vi "AWG Start Pulses.vi"(8 "error in (no error)":errorcluster, 10 "T [s] (1ms)":dbl=0.001, 11 "awg session in":T1) -> (0 "error out":errorcluster, 3 "awg session out":T1)   [LabVIEW 2013, in "AWG.lvlib"]
doc: "AWG wrapper: Starts infinite pulse train with given period."
uses:
  AWG.lvlib
  AWG Session.ctl
  AWG Type.ctl
  Agilent 33XXX Series/Agilent 33XXX Series.lvlib
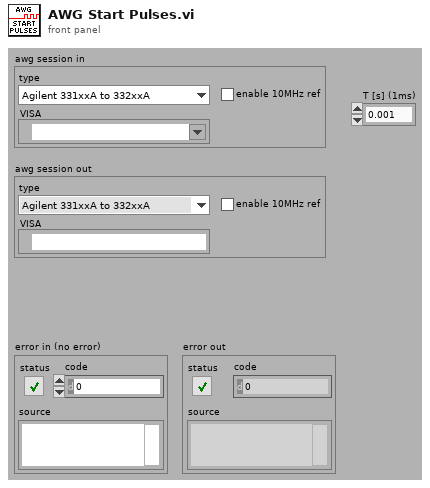
[diagram p1: front panel]
types:
  T1 = typedef "AWG.lvlib/AWG Session.ctl" = cluster{"type":T2, "VISA":refnum<visa-resource-name>, "enable 10MHz ref":bool}
  T2 = typedef "AWG.lvlib/AWG Type.ctl" = enum16{"Agilent 331xxA to 332xxA", "Agilent 335xxA to 336xxA", "dummy"}
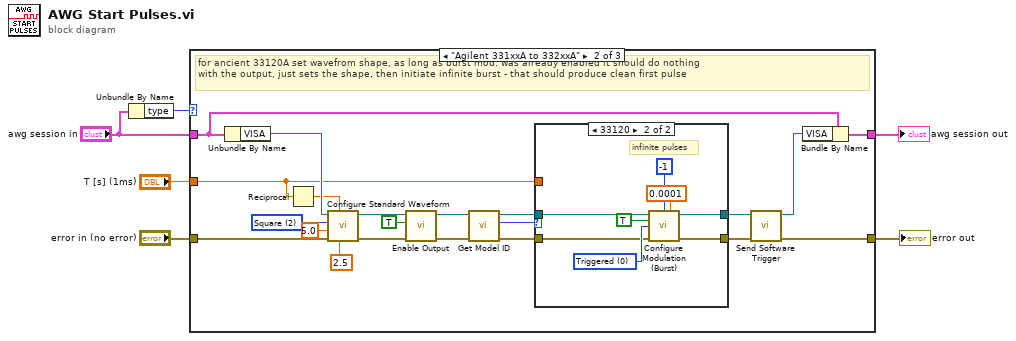
[diagram p0: block diagram]
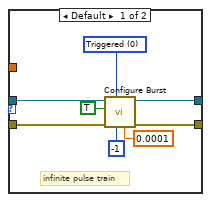
[diagram p3: hidden frame]
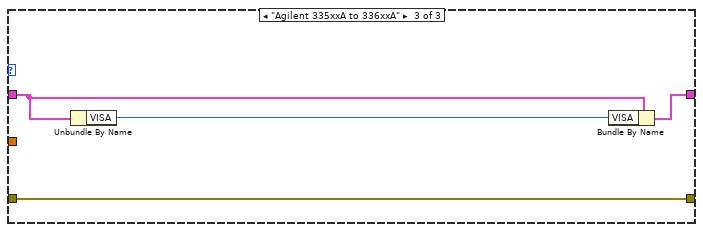
[diagram p4: hidden frame]
diagram:
  n1 = Unbundle By Name("awg session in") -> ("type"=w6:T2)
  n2 = case shown="\"Agilent 331xxA to 332xxA\"" w6 {
    tunnel: "error in (no error)" -> [w8 w20 w46]
    tunnel: [w8 w27 w46] -> w4
    tunnel: "awg session in" -> [w7 w28 w49]
    tunnel: [w7 w29 w48] -> w2
    tunnel: "T [s] (1ms)" -> [_ w9 _]
    frame Default {
    }
    frame "Agilent 331xxA to 332xxA" {
      w23 = u16 2 items=["DC", "Sine", "Square", "Triangle", "Ramp", "Pulse", "Noise", "Sinc", "Negative Ramp", "Exponential Rise", "Exponential Fall", "Cardiac"] ("Waveform Function (1: Sine)")
      # "for ancient 33120A set wavefrom shape, as long as burst mod. was already enabled it should do nothing\nwith the output, just sets the shape, then initiate infinite burst - that should produce clean first pulse"
      n3 = Unbundle By Name(w28) -> ("VISA"=w21:refnum<visa-resource-name>)
      n4 = Reciprocal(x=w9) -> (1/x=w10:dbl)
      n5 = call "Configure Standard Waveform.vi"("DC Offset (0.00 V)"=2.5, "Frequency (1000 Hz)"=w10, "error in (no error)"=w20, "Amplitude (1)"=5.0, "Waveform Function (1: Sine)"=w23, "VISA resource name"=w21) -> ("error out"=w18:errorcluster, "VISA resource name out"=w17:refnum<visa-resource-name>)  [unwired: 4 in]
      n6 = call "Enable Output.vi"("error in (no error)"=w18, "Enable Output  (T: Enable)"=TRUE, "VISA resource name"=w17) -> ("error out"=w15:errorcluster, "VISA resource name out"=w14:refnum<visa-resource-name>)  [unwired: 7 in]
      n7 = call "Get Model ID.vi"("error in (no error)"=w15, "VISA resource name"=w14) -> ("error out"=w13:errorcluster, "model ID"=w12:u32, "VISA resource name out"=w11:refnum<visa-resource-name>)  [unwired: 7 in]
      n8 = case shown="33120" w12 {
        tunnel: [w36 w42] -> w25
        tunnel: [w35 w41] -> w24
        tunnel: w9 -> [_ _]
        tunnel: w13 -> [w37 w40]
        tunnel: w11 -> [w34 w39]
        frame Default {
          w33 = u16 0 items=["Triggered", "Gated"] ("Burst Mode (0: Triggered)")
          # "infinite pulse train"
          n9 = call "Configure Burst.vi"("Burst Period (1 s)"=0.0001, "Burst Count (1)"=-1, "Burst Mode (0: Triggered)"=w33, "error in (no error)"=w37, "Enable Burst (T: Enable)"=TRUE, "VISA resource name"=w34) -> ("error out"=w36:errorcluster, "VISA resource name out"=w35:refnum<visa-resource-name>)  [unwired: 4 in]
        }
        frame 33120 {
          w43 = u16 0 items=["Triggered", "Gated"] ("Burst Modulation Mode (0: Triggered)")
          # "infinite pulses"
          n10 = call "Configure Modulation (Burst).vi"("VISA resource name"=w39, "Burst Count (1)"=-1, "Burst Period (1 s)"=0.0001, "Enable Burst Modulation (T: Enable)"=TRUE, "Burst Modulation Mode (0: Triggered)"=w43, "error in (no error)"=w40) -> ("VISA resource name out"=w41:refnum<visa-resource-name>, "error out"=w42:errorcluster)  [unwired: 8 in]
        }
      }
      n11 = call "Send Software Trigger.vi"("error in (no error)"=w25, "VISA resource name"=w24) -> ("error out"=w27:errorcluster, "VISA resource name out"=w26:refnum<visa-resource-name>)  [unwired: 8 in]
      n12 = Bundle By Name(cluster=w28, "VISA"=w26) -> (w29:T1)
    }
    frame "Agilent 335xxA to 336xxA" {
      n13 = Unbundle By Name(w49) -> ("VISA"=w47:refnum<visa-resource-name>)
      n14 = Bundle By Name(cluster=w49, "VISA"=w47) -> (w48:T1)
    }
  }
  "error out" <- w4
  "awg session out" <- w2
